vi "Get Log File Reference.vi"(8 "Error In":errorcluster, 11 "Error Handling In":refnum<class "Error Handling.lvclass">) -> (0 "Error Out":errorcluster, 2 "Log File Reference":refnum<file>, 3 "Error Handling Out":refnum<class "Error Handling.lvclass">)   [LabVIEW 2021, in "Error Handling.lvclass"]
uses:
  Error Handling.lvclass
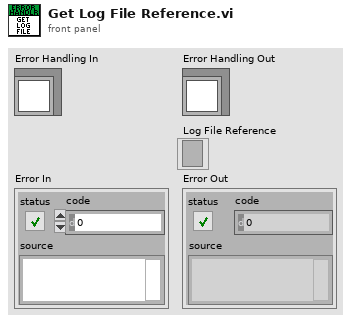
[diagram p1: front panel]
types:
  T1 = typedef "Error Handling.lvclass/Data.ctl" = cluster{"Log File Reference":refnum<file>}
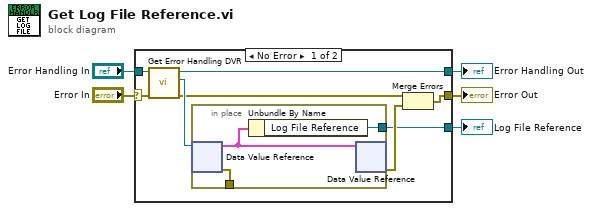
[diagram p0: block diagram]
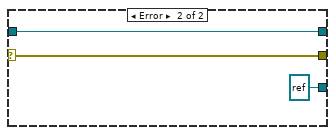
[diagram p2: hidden frame]
diagram:
  n1 = case shown="No Error" "Error In" {
    selector: "Error In" -> [w9 w18]
    tunnel: [w11 w18] -> w2
    tunnel: [w8 w19] -> w4
    tunnel: "Error Handling In" -> [w10 w19]
    tunnel: [w12 refnum<file> refnum ("Log File Reference")] -> w1
    frame No Error {
      n2 = call "Get Error Handling DVR.vi"("Error In"=w9, "Error Handling In"=w10) -> ("Error Out"=w6:errorcluster, "DVR"=w7:refnum<data-value>, "Error Handling Out"=w8:refnum<class "Error Handling.lvclass">)  [unwired: 7 in]
      n3 = in-place {
        in-place-border: [w14] -> w12
        in-place-border: [w16] -> _
        n4 = in-place-dvr #1(w7) -> (w15:T1, w16:errorcluster)
        n5 = Unbundle By Name(w15) -> ("Log File Reference"=w14:refnum<file>)
        n6 = in-place-dvr #1(w15) -> (w13:errorcluster)  [unwired: 1 out]
      }
      n7 = Merge Errors(w6, w13) -> (w11:errorcluster)
    }
    frame Error {
    }
  }
  "Error Handling Out" <- w4
  "Error Out" <- w2
  "Log File Reference" <- w1
